vi "Inline - Update Error Counters Channels_Increment Counter and Update NI-VSChannel.vi"(8 "error in (no error)":errorcluster, 9 "Inline Status Channels Refs":T1[](array[typedef]) format="%.0x", 10 "index":i32, 11 "Error Counters Value In in":u32[](array[numeric])) -> (0 "error out":errorcluster, 3 "Error Counters Value In out":u32[](array[numeric]))   [LabVIEW 2020, in "Ballard Arinc-429 Engine.lvlib"]
uses:
  Ballard Arinc-429 Engine.lvlib
  <vilib>/NI VeriStand/Custom Device API/Data Reference.ctl
  RT Controls/Inline_Status_Channels.ctl
  <vilib>/NI VeriStand/Custom Device API/Global Data Refs.vi
  <vilib>/NI VeriStand/Custom Device API/Custom Device API.lvlib
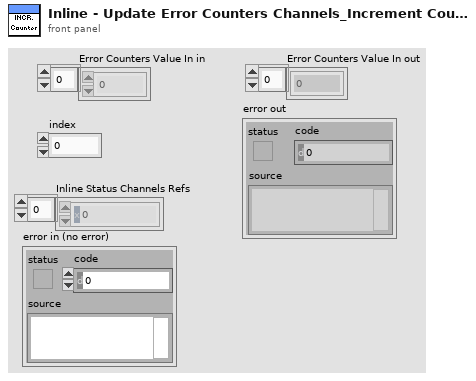
[diagram p1: front panel]
types:
  T1 = typedef "Custom Device API.lvlib/Data Reference.ctl" = i32
  T2 = typedef "Ballard Arinc-429 Engine.lvlib/Inline_Status_Channels.ctl" = enum16{"Error Code", "Inline Read Time (us)", "Inline Write Time (us)", "Receiving Error - Error Counter", "Gap Error - Error Counter", "Parity Error - Error Counter", "Long Word Error - Error Counter", "Bit Timing Error - Error Counter"}
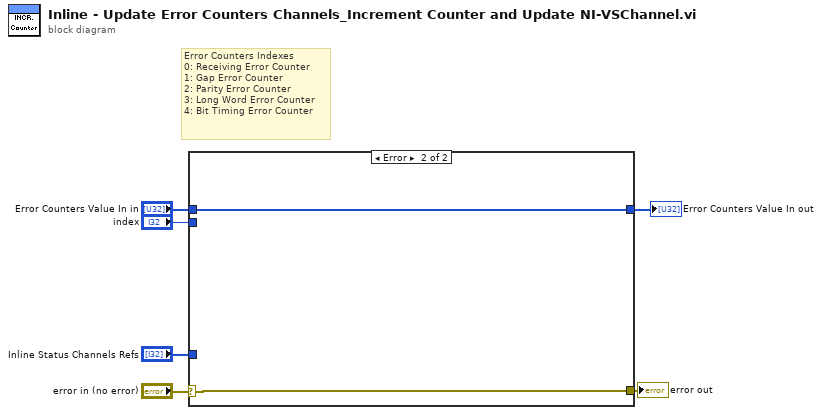
[diagram p0: block diagram]
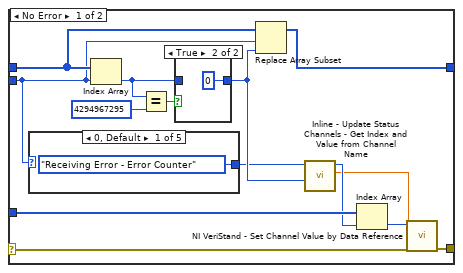
[diagram p2: hidden frame]
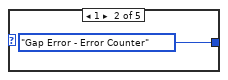
[diagram p3: hidden frame]
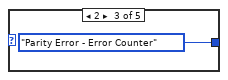
[diagram p4: hidden frame]
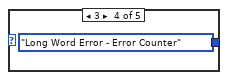
[diagram p5: hidden frame]
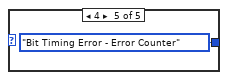
[diagram p6: hidden frame]
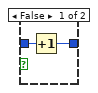
[diagram p7: hidden frame]
diagram:
  # "Error Counters Indexes\n0: Receiving Error Counter\n1: Gap Error Counter\n2: Parity Error Counter\n3: Long Word Error Counter\n4: Bit Timing Error Counter"
  n1 = case shown="Error" "error in (no error)" {
    selector: "error in (no error)" -> [w7 w30]
    tunnel: [w20 w29] -> w6
    tunnel: "Error Counters Value In in" -> [w16 w29]
    tunnel: "Inline Status Channels Refs" -> [w14 _]
    tunnel: "index" -> [w12 _]
    tunnel: [w8 w30] -> w2
    frame No Error {
      n2 = case shown="0, Default" w12 {
        tunnel: [Inline_Status_Channels."Receiving Error - Error Counter" ("Status Channel") Inline_Status_Channels."Gap Error - Error Counter" ("Status Channel") Inline_Status_Channels."Parity Error - Error Counter" ("Status Channel") Inline_Status_Channels."Long Word Error - Error Counter" ("Status Channel") Inline_Status_Channels."Bit Timing Error - Error Counter" ("Status Channel")] -> w11
        frame 0, Default {
        }
        frame 1 {
        }
        frame 2 {
        }
        frame 3 {
        }
        frame 4 {
        }
      }
      n3 = Index Array(array=w16, index=w12) -> (element=w19:u32)
      n4 = Equal?(x=w19, y=u32 4294967295) -> (x = y?=w18:bool)
      n5 = case shown="True" w18 {
        tunnel: w19 -> [w27 _]
        tunnel: [w26 u32 0] -> w15
        frame False {
          n6 = Increment(x=w27) -> (x+1=w26:u32)
        }
        frame True {
        }
      }
      n7 = Replace Array Subset(array=w16, new element=w15, index=w12) -> (w20:u32[])
      n8 = call "Inline - Update Status Channels - Get Index and Value from Channel Name.vi"("Time (us)/Error Counter Value"=w15, "Status Channel"=w11) -> ("Value"=w9:dbl, "index"=w13:i32)  [unwired: 8 in]
      n9 = Index Array(array=w14, index=w13) -> (element=w10:T1)
      n10 = call <vilib>:"NI VeriStand - Set Channel Value by Data Reference.vi"("error in (no error)"=w7, "Value"=w9, "Data Reference in"=w10) -> ("error out"=w8:errorcluster)  [unwired: 8 in]
    }
    frame Error {
    }
  }
  "Error Counters Value In out" <- w6
  "error out" <- w2
